vi "SetClearCycles.vi"(6 "CC Max":refnum<vi>, 9 "CC Min":refnum<vi>, 10 "Clear Cycle":refnum<vi>, 11 ".NET Refnum in":refnum<k24>) -> ()   [LabVIEW 2018]
uses:
  D:/SVN/PM/sdk/AppSamples/LabVIEWSamples/trunk/Release/2018/Dependencies/PVCamNET.dll
  Dependencies/PVCamNET.dll
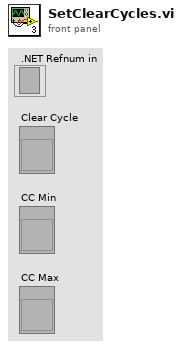
[diagram p1: front panel]
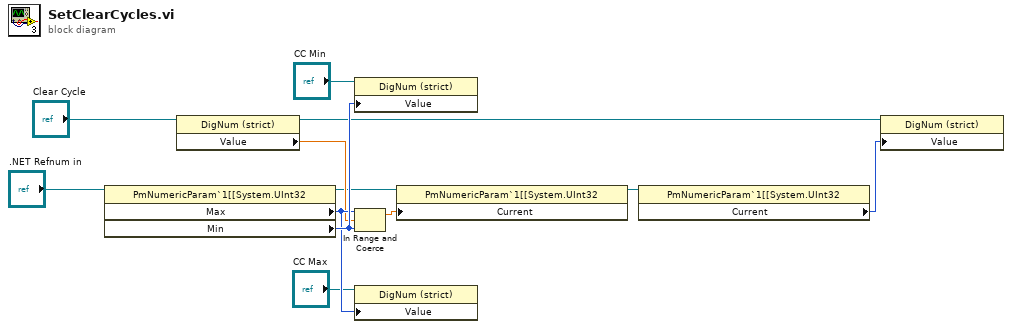
[diagram p0: block diagram]
diagram:
  n1 = property class="PmNumericParam`1[[System.UInt32"(reference=".NET Refnum in") -> (reference out=w2:refnum<k24>, "Max"=w11:u32, "Min"=w12:u32)  [unwired: 1 in, 1 out]
  n2 = property class="DigNum (strict)"(reference="Clear Cycle") -> (reference out=w6:refnum<vi>, "Value"=w7:dbl)  [unwired: 1 in, 1 out]
  n3 = property class="DigNum (strict)"(reference="CC Min", "Value"=w12) -> ()  [unwired: 1 in, 2 out]
  n4 = In Range and Coerce(upper limit=w11, x=w7, lower limit=w12) -> (coerced(x)=w3:dbl)  [unwired: 1 out]
  n5 = property class="DigNum (strict)"(reference="CC Max", "Value"=w11) -> ()  [unwired: 1 in, 2 out]
  n6 = property class="PmNumericParam`1[[System.UInt32"(reference=w2, "Current"=w3) -> (reference out=w4:refnum<k24>)  [unwired: 1 in, 1 out]
  n7 = property class="PmNumericParam`1[[System.UInt32"(reference=w4) -> ("Current"=w8:u32)  [unwired: 1 in, 2 out]
  n8 = property class="DigNum (strict)"(reference=w6, "Value"=w8) -> ()  [unwired: 1 in, 2 out]
